vi "ConsolidatedLimitSwitchMotors.vi"(8 "CurrentLSValue":bool, 9 "LastLSValue":bool, 10 "CurrentInput":dbl, 11 "LastSign":dbl) -> (0 "New Output":dbl, 3 "NewSign":dbl)   [LabVIEW 2012]
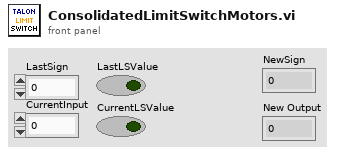
[diagram p1: front panel]
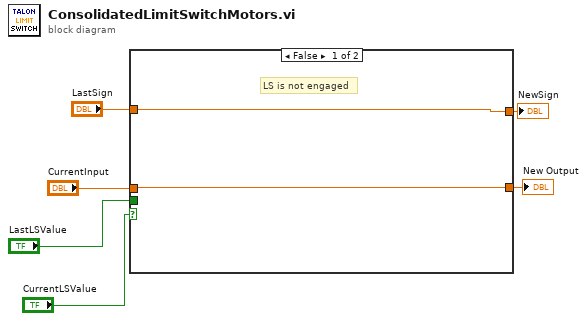
[diagram p0: block diagram]
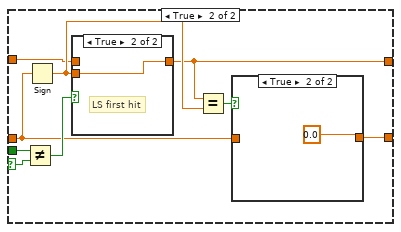
[diagram p2: hidden frame]
diagram:
  n1 = case shown="False" "CurrentLSValue" {
    selector: "CurrentLSValue" -> [_ w17]
    tunnel: "CurrentInput" -> [w7 w9]
    tunnel: [w7 w12] -> w1
    tunnel: "LastLSValue" -> [_ w16]
    tunnel: "LastSign" -> [w8 w11]
    tunnel: [w8 w10] -> w2
    frame False {
      # "LS is not engaged"
    }
    frame True {
      n2 = Not Equal?(x=w16, y=w17) -> (x != y?=w15:bool)
      n3 = Sign(1:w9) -> (0:w14:dbl)
      n4 = case shown="True" w15 {
        tunnel: w11 -> [w20 _]
        tunnel: w14 -> [_ w21]
        tunnel: [w20 w21] -> w10
        frame False {
          # "LS is still\nengaged"
        }
        frame True {
          # "LS first hit"
        }
      }
      n5 = Equal?(x=w10, y=w14) -> (x = y?=w13:bool)
      n6 = case shown="True" w13 {
        tunnel: [w18 0.0] -> w12
        tunnel: w9 -> [w18 _]
        frame False {
        }
        frame True {
        }
      }
    }
  }
  "NewSign" <- w2
  "New Output" <- w1
